vi "Fit Pitch Axis(SubVI).vi"(8 "error in (no error)":errorcluster, 11 "Array of Joint Positions in":dbl[][](array[numeric])) -> (0 "error out":errorcluster, 3 "Pitch":dbl)   [LabVIEW 2014]
uses:
  <vilib>/Analysis/NI_AALPro.lvlib
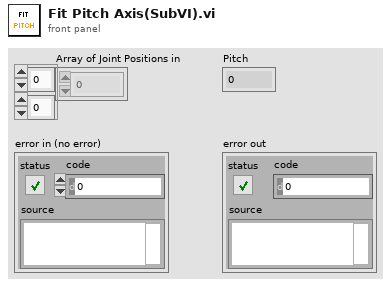
[diagram p1: front panel]
types:
  T1 = enum16{"hip centre", "spine", "shoulder centre", "head", "shoulder left", "elbow left", "wrist left", "hand left", "shoulder right", "elbow right", "wrist right", "hand right", "hip left", "knee left", "ankle left", "foot left", "hip right", "knee right", "ankle right", "foot right"}
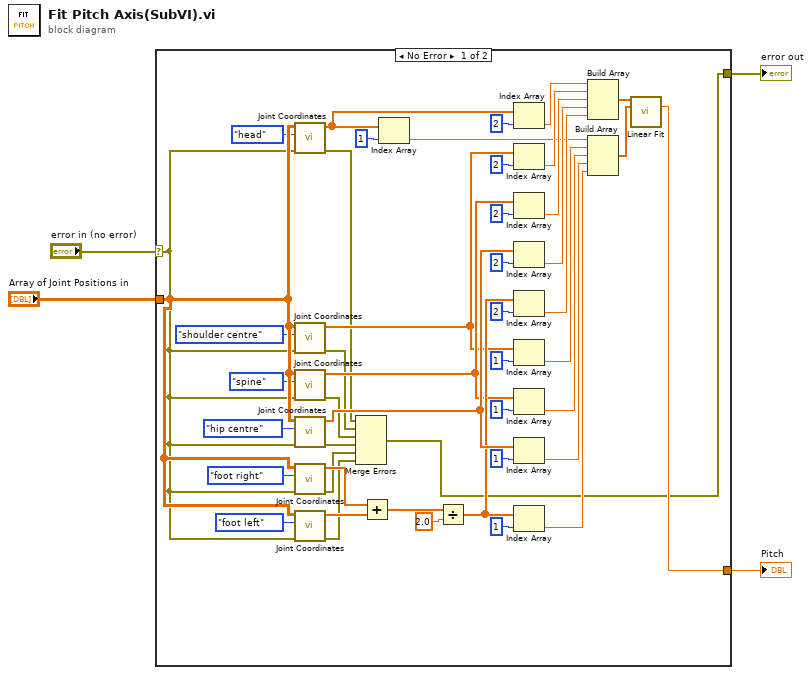
[diagram p0: block diagram]
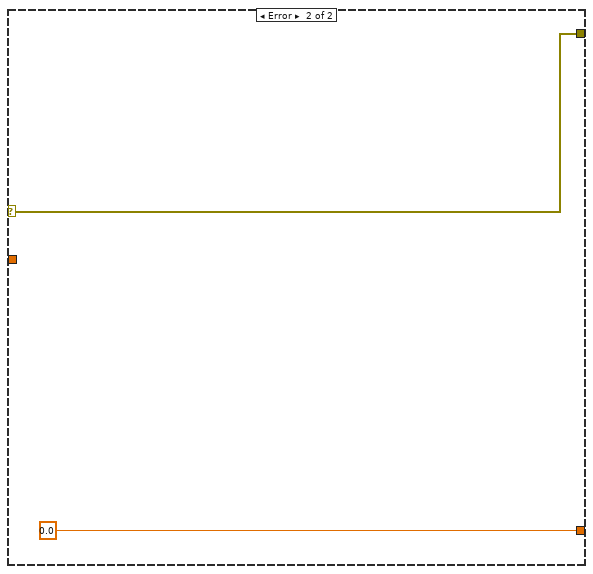
[diagram p2: hidden frame]
diagram:
  n1 = case shown="No Error" "error in (no error)" {
    selector: "error in (no error)" -> [w5 w53]
    tunnel: "Array of Joint Positions in" -> [w51 _]
    tunnel: [w49 0.0 ("slope")] -> w3
    tunnel: [w33 w53] -> w2
    frame No Error {
      n2 = call <vilib>:"Joint Coordinates.vi"("error in (no error)"=w5, "Joint 1"=T1."head", "Array of Joint Positions"=w51) -> ("error out"=w6:errorcluster, "Joint Coordinates"=w18:dbl[])  [unwired: 7 in]
      n3 = call <vilib>:"Joint Coordinates.vi"("error in (no error)"=w5, "Joint 1"=T1."shoulder centre", "Array of Joint Positions"=w51) -> ("error out"=w7:errorcluster, "Joint Coordinates"=w19:dbl[])  [unwired: 7 in]
      n4 = call <vilib>:"Joint Coordinates.vi"("error in (no error)"=w5, "Joint 1"=T1."spine", "Array of Joint Positions"=w51) -> ("error out"=w8:errorcluster, "Joint Coordinates"=w20:dbl[])  [unwired: 7 in]
      n5 = call <vilib>:"Joint Coordinates.vi"("error in (no error)"=w5, "Joint 1"=T1."hip centre", "Array of Joint Positions"=w51) -> ("error out"=w9:errorcluster, "Joint Coordinates"=w50:dbl[])  [unwired: 7 in]
      n6 = call <vilib>:"Joint Coordinates.vi"("error in (no error)"=w5, "Joint 1"=T1."foot right", "Array of Joint Positions"=w51) -> ("error out"=w34:errorcluster, "Joint Coordinates"=w40:dbl[])  [unwired: 7 in]
      n7 = call <vilib>:"Joint Coordinates.vi"("error in (no error)"=w5, "Joint 1"=T1."foot left", "Array of Joint Positions"=w51) -> ("error out"=w35:errorcluster, "Joint Coordinates"=w41:dbl[])  [unwired: 7 in]
      n8 = Merge Errors(w6, w7, w8, w9, w34, w35) -> (w33:errorcluster)
      n9 = Add(x=w40, y=w41) -> (x+y=w39:dbl[])
      n10 = Index Array(array=w18, index=1) -> (element=w21:dbl)
      n11 = Divide(x=w39, y=2.0) -> (x/y=w44:dbl[])
      n12 = Index Array(array=w18, index=2) -> (element=w25:dbl)
      n13 = Index Array(array=w19, index=2) -> (element=w26:dbl)
      n14 = Index Array(array=w20, index=2) -> (element=w27:dbl)
      n15 = Index Array(array=w50, index=2) -> (element=w28:dbl)
      n16 = Index Array(array=w44, index=2) -> (element=w45:dbl)
      n17 = Index Array(array=w19, index=1) -> (element=w22:dbl)
      n18 = Index Array(array=w20, index=1) -> (element=w23:dbl)
      n19 = Index Array(array=w50, index=1) -> (element=w24:dbl)
      n20 = Index Array(array=w44, index=1) -> (element=w46:dbl)
      n21 = Build Array(w25, w26, w27, w28, w45) -> (w47:dbl[])
      n22 = Build Array(w21, w22, w23, w24, w46) -> (w48:dbl[])
      n23 = call <vilib>:"Linear Fit.vi"("Y"=w47, "X"=w48) -> ("slope"=w49:dbl)  [unwired: 9 in, 4 out]
    }
    frame Error {
    }
  }
  "Pitch" <- w3
  "error out" <- w2
